vi "Laser Control.vi"(10 "Trial In Progress IN":T1, 11 "Trial Fraction IN":dbl) -> (0 "Laser Trig Analog Output":dbl, 1 "laser_ctrl":bool, 2 "Laser Pulse OFF Time (msec)":i16, 3 "Laser Pulse ON Time (msec)":i16)   [LabVIEW 2018]
uses:
  controls/Trial Config Settings.ctl
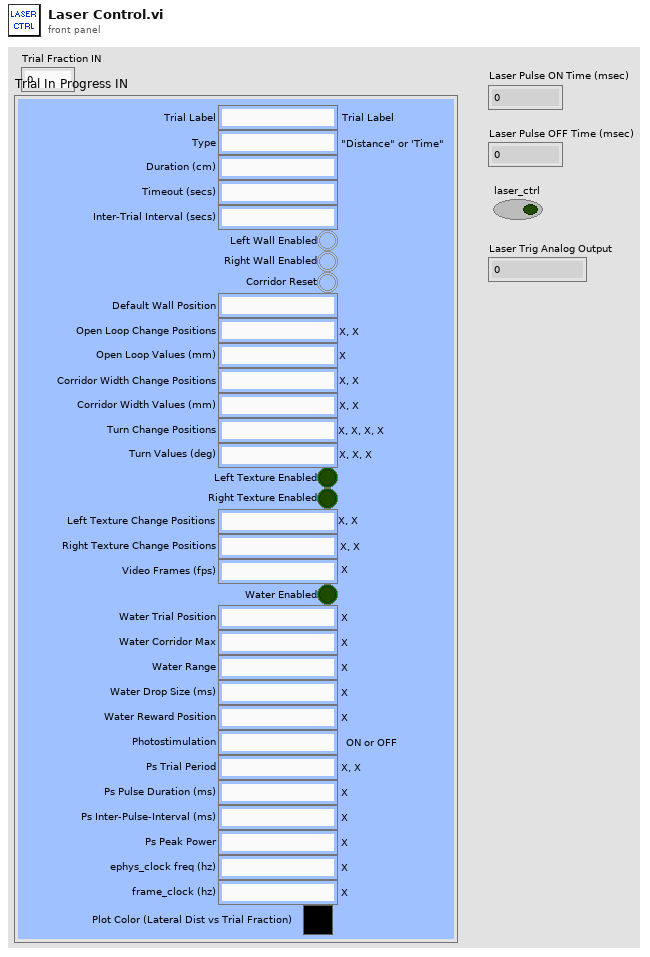
[diagram p1: front panel]
types:
  T1 = typedef "Trial Config Settings.ctl" = cluster{"Trial Label":string, "Type":string, "Timeout (secs)":string, "Inter-Trial Interval (secs)":string, "Left Wall Enabled":bool, "Right Wall Enabled":bool, "Corridor Reset":bool, "Default Wall Position":string, "Open Loop Change Positions":string, "Open Loop Values (mm)":string, "Corridor Width Change Positions":string, "Corridor Width Values (mm) ":string, "Turn Change Positions":string, "Turn Values (deg)":string, "Left Texture Change Positions":string, "Right Texture Change Positions":string, "Video Frames (fps)":string, "Water Enabled":bool, "Water Trial Position":string, "Photostimulation":string, "Water Corridor Max":string, "Water Range":string, "Water Drop Size (ms)":string, "Water Reward Position":string, "Duration (cm)":string, "Left Texture Enabled":bool, "Right Texture Enabled":bool, "Ps Trial Period":string, "Ps Inter-Pulse-Interval (ms)":string, "Ps Peak Power":string, "Ps Pulse Duration (ms)":string, "ephys_clock freq (hz)":string, "frame_clock (hz)":string, "Plot Color (Lateral Dist vs Trial Fraction)":u32}
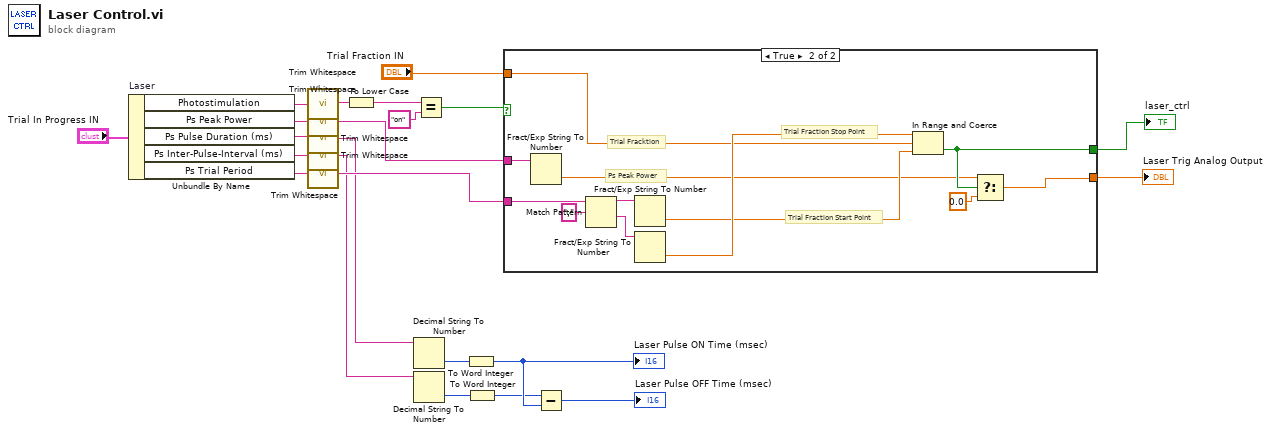
[diagram p0: block diagram]
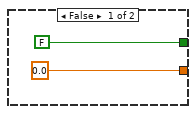
[diagram p2: hidden frame]
diagram:
  n1 = Unbundle By Name "Laser"("Trial In Progress IN") -> ("Photostimulation"=w7:string, "Ps Peak Power"=w10:string, "Ps Pulse Duration (ms)"=w16:string, "Ps Inter-Pulse-Interval (ms)"=w17:string, "Ps Trial Period"=w19:string)
  n2 = call <vilib>:"Trim Whitespace.vi"("string"=w7) -> ("trimmed string"=w6:string)  [unwired: 1 in]
  n3 = call <vilib>:"Trim Whitespace.vi"("string"=w10) -> ("trimmed string"=w11:string)  [unwired: 1 in]
  n4 = call <vilib>:"Trim Whitespace.vi"("string"=w16) -> ("trimmed string"=w15:string)  [unwired: 1 in]
  n5 = call <vilib>:"Trim Whitespace.vi"("string"=w17) -> ("trimmed string"=w14:string)  [unwired: 1 in]
  n6 = call <vilib>:"Trim Whitespace.vi"("string"=w19) -> ("trimmed string"=w20:string)  [unwired: 1 in]
  n7 = To Lower Case(string=w6) -> (all lower case string=w8:string)
  n8 = Decimal String To Number(string=w15) -> (number=w4:i32)  [unwired: 2 in, 1 out]
  n9 = Decimal String To Number(string=w14) -> (number=w2:i32)  [unwired: 2 in, 1 out]
  n10 = Equal?(x=w8, y="on") -> (x = y?=w9:bool)
  n11 = To Word Integer(number=w4) -> (16bit integer=w3:i16)
  "Laser Pulse ON Time (msec)" <- w3
  n12 = To Word Integer(number=w2) -> (16bit integer=w1:i16)
  n13 = case shown="True" w9 {
    tunnel: [FALSE w28] -> w13
    tunnel: w20 -> [_ w29]
    tunnel: "Trial Fraction IN" -> [_ w31]
    tunnel: w11 -> [_ w30]
    tunnel: [0.0 w26] -> w12
    frame False {
    }
    frame True {
      # "Trial Fraction Stop Point"
      # "Trial Fraction Start Point"
      # "Ps Peak Power"
      # "Trial Fracktion"
      n14 = Fract/Exp String To Number(string=w30) -> (number=w27:dbl)  [unwired: 3 in, 1 out]
      n15 = Match Pattern(string=w29, regular expression=",") -> (before substring=w36:string, after substring=w35:string)  [unwired: 1 in, 2 out]
      n16 = Fract/Exp String To Number(string=w36) -> (number=w32:dbl)  [unwired: 3 in, 1 out]
      n17 = Fract/Exp String To Number(string=w35) -> (number=w33:dbl)  [unwired: 3 in, 1 out]
      n18 = In Range and Coerce(upper limit=w33, x=w31, lower limit=w32) -> (In Range?=w28:bool)  [unwired: 1 out]
      n19 = Select(t=w27, s=w28, f=0.0) -> (s? t:f=w26:dbl)
    }
  }
  "laser_ctrl" <- w13
  "Laser Trig Analog Output" <- w12
  n20 = Subtract(x=w1, y=w3) -> (x-y=→"Laser Pulse OFF Time (msec)":i16)
